vi "CheckifVeriStandisRunning.vi"(8 "error in (no error)":errorcluster) -> (0 "error out":errorcluster, 3 "VeriStand Running":bool)   [LabVIEW 2017, in "VeriStandTestUtilities.lvlib"]
uses:
  VeriStandTestUtilities.lvlib
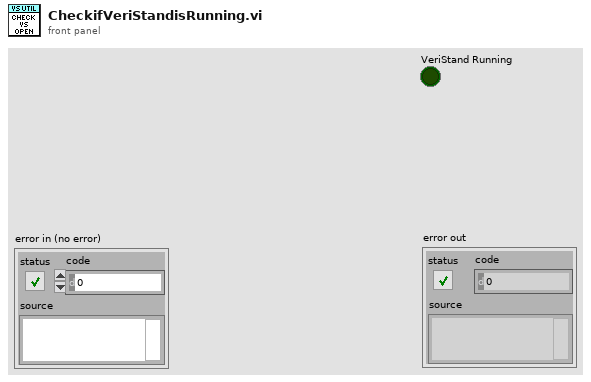
[diagram p1: front panel]
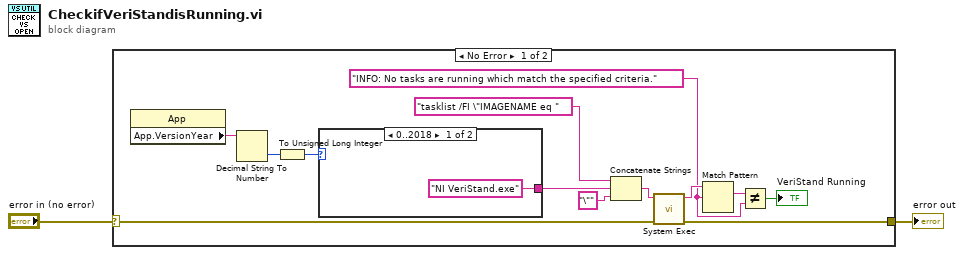
[diagram p0: block diagram]
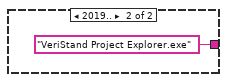
[diagram p2: hidden frame]
diagram:
  n1 = case shown="No Error" "error in (no error)" {
    selector: "error in (no error)" -> [w4 w18]
    tunnel: [w3 w18] -> w1
    frame No Error {
      w7 = "INFO: No tasks are running which match the specified criteria."
      n2 = property class="App"() -> ("App.VersionYear"=w14:string)  [unwired: 2 in, 2 out]
      n3 = Decimal String To Number(string=w14) -> (number=w15:i32)  [unwired: 2 in, 1 out]
      n4 = To Unsigned Long Integer(number=w15) -> (unsigned 32bit integer=w13:u32)
      n5 = case shown="0..2018" w13 {
        tunnel: ["NI VeriStand.exe" ("command line") "VeriStand Project Explorer.exe" ("command line")] -> w9
        frame 0..2018 {
        }
        frame 2019.. {
        }
      }
      n6 = Concatenate Strings("tasklist /FI \"IMAGENAME eq ", w9, "\"" ("string")) -> (w11:string)
      n7 = call <vilib>:"System Exec.vi"("error in (no error)"=w4, "command line"=w11) -> ("error out"=w3:errorcluster, "standard output"=w8:string)  [unwired: 6 in, 2 out]
      n8 = Match Pattern(string=w8, regular expression=w7) -> (match substring=w6:string)  [unwired: 1 in, 3 out]
      n9 = Not Equal?(x=w6, y=w7) -> (x != y?=→"VeriStand Running":bool)
    }
    frame Error {
    }
  }
  "error out" <- w1
